vi "2022.09.08视觉菜鸟.vi"(7 "error in":errorcluster) -> (27 "error out":errorcluster)   [LabVIEW 2018]
uses:
  <vilib>/vision/NI_Vision_Development_Module.lvlib
panel:
  out "Image Out":T1(plugin-control)
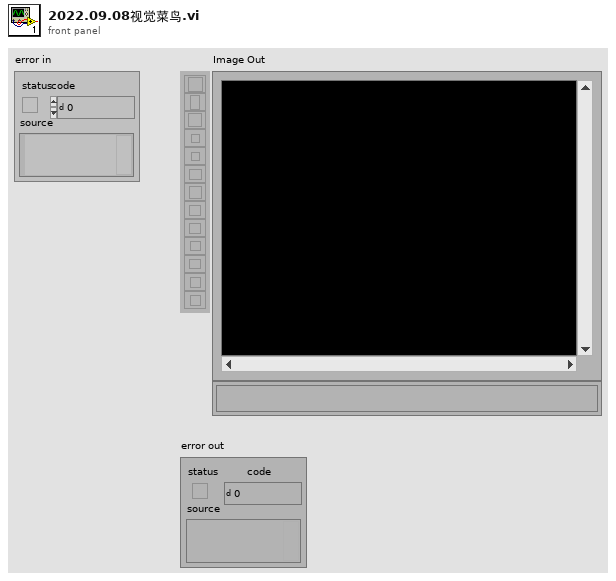
[diagram p1: front panel]
types:
  T1 = typedef "IMAQ Image.ctl" = refnum<image>
  T2 = cluster{"Brightness":sgl, "Contrast":sgl, "Gamma":sgl}
  T3 = typedef "Image Type" = u32
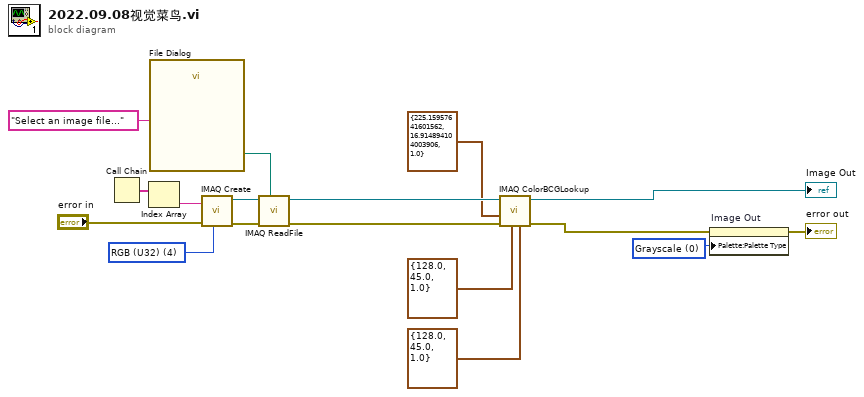
[diagram p0: block diagram]
diagram:
  w1 = u32 0 items=["Grayscale", "Binary", "Gradient", "Rainbow", "Temperature", "User Defined", "Binary 16 Bit", "Gradient 16 Bit", "Rainbow 16 Bit", "Temperature 16 Bit", "User Defined 16 Bit"] ("Palette Type")
  w9 = T3 4 items=["Grayscale (U8)", "Grayscale (I16)", "Grayscale (SGL)", "Complex (CSG)", "RGB (U32)", "HSL (U32)", "RGB (U64)", "Grayscale (U16)"] ("Image Type")
  n1 = Call Chain() -> (call chain=w13:string[])
  n2 = Index Array(array=w13) -> (element=w12:string)  [unwired: 1 in]
  n3 = call "File Dialog"("prompt"="Select an image file...") -> ("selected path"=w10:path)  [unwired: 6 in, 8 out]
  n4 = call "IMAQ Create"("Image Name"=w12, "Image Type"=w9, "error in (no error)"="error in") -> ("New Image"=w16:T1, "error out"=w15:errorcluster)  [unwired: 1 in, 1 out]
  n5 = call "IMAQ ReadFile"("File Path"=w10, "error in (no error)"=w15, "Image"=w16) -> ("error out"=w17:errorcluster, "Image Out"=w8:T1)  [unwired: 2 in, 5 out]
  n6 = call "IMAQ ColorBCGLookup"("Blue BCG Values"=T2 {"Brightness"=128.0, "Contrast"=45.0, "Gamma"=1.0}, "Green BCG Values"=T2 {"Brightness"=128.0, "Contrast"=45.0, "Gamma"=1.0}, "error in (no error)"=w17, "Red BCG Values"=T2 {"Brightness"=225.15958, "Contrast"=16.914894, "Gamma"=1.0}, "Image Src"=w8) -> ("error out"=w7:errorcluster, "Image Dst Out"=→"Image Out":T1)  [unwired: 2 in, 3 out]
  n7 = property on="Image Out" class="ImageControl"(error in=w7, "Palette:Palette Type"=w1) -> (error out=→"error out":errorcluster)  [unwired: 1 in, 1 out]
